vi "Most Recent Distance Traveled.vi"(7 "Set or Get Value":enum16{"Set", "Get"}(ring), 8 "error in":errorcluster, 11 "Distance":i32) -> (0 "error out":errorcluster, 3 "Saved Distance":i32)   [LabVIEW 2009, in "Sliding Menu Library.lvlib"]
uses:
  Sliding Menu Library.lvlib
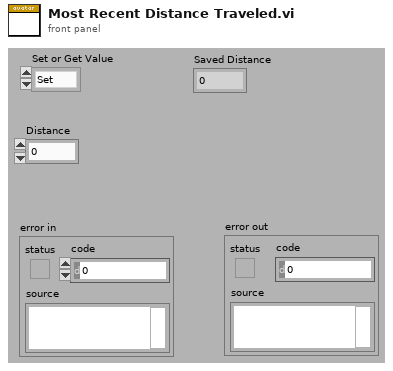
[diagram p1: front panel]
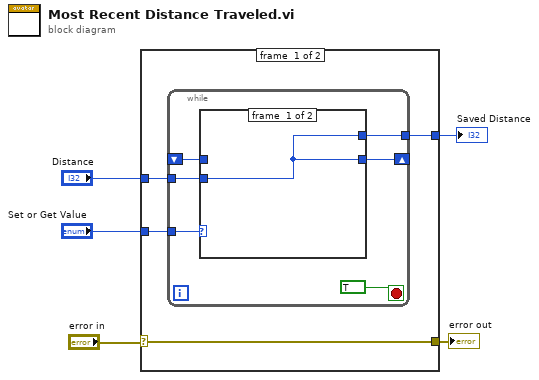
[diagram p0: block diagram]
diagram:
  n1 = case shown="No Error" "error in" {
    selector: "error in" -> [w7 w19]
    tunnel: "Set or Get Value" -> [w9 _]
    tunnel: "Distance" -> [w8 _]
    tunnel: [w7 w19] -> w2
    tunnel: [w6 _] -> w1
    frame #0 {
      n2 = while {
        tunnel: w8 -> [w14]
        shift-right: [w11] -> _
        shift-left: _ -> [w13]
        tunnel: w9 -> [w12]
        tunnel: [w10] -> w6
        stop <- TRUE stop-if-true
        n3 = case shown="\"Get\", Default" w12 {
          tunnel: w14 -> [w16 w17]
          tunnel: [w16 w17] -> w11
          tunnel: w13 -> [_ w18]
          tunnel: [w16 w18] -> w10
          frame #0 {
          }
          frame #1 {
          }
        }
      }
    }
    frame #1 {
    }
  }
  "Saved Distance" <- w1
  "error out" <- w2
